vi "Close Doors.vi"(8 "error in (no error)":errorcluster, 11 "Door Hardware in":refnum<class "Door Hardware.lvclass">) -> (0 "error out":errorcluster, 3 "Door Hardware out":refnum<class "Door Hardware.lvclass">)   [LabVIEW 2020, in "Door Hardware.lvlib" / "Door Hardware.lvclass"]
uses:
  Door Hardware.lvclass
  Door Hardware.lvclass/Door Hardware.ctl
  Door Actuator/Door Actuator.lvclass
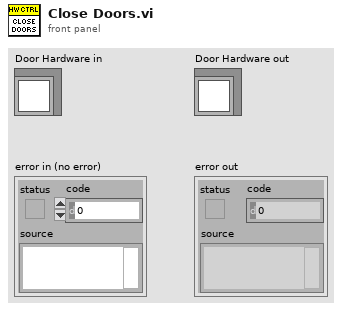
[diagram p1: front panel]
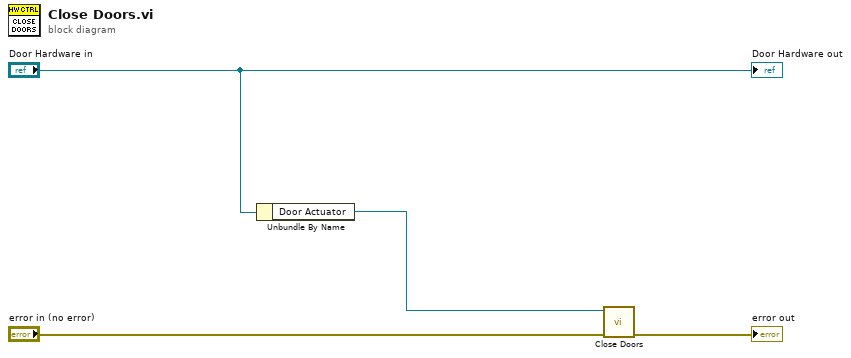
[diagram p0: block diagram]
diagram:
  n1 = Unbundle By Name("Door Hardware in") -> ("Door Actuator"=w3:refnum<class "Door Actuator.lvclass">)
  n2 = call-dynamic "Close Doors.vi"("error in (no error)"="error in (no error)", "Door Actuator in"=w3) -> ("error out"=→"error out":errorcluster)  [unwired: 8 in, 1 out]
  "Door Hardware out" <- "Door Hardware in"
